vi "TidyOverlappingWiresSubVi.vi"(8 "Error In":errorcluster, 10 "Control references":refnum<vi>[](array[refnum]), 11 "New case structure ref":refnum<vi>) -> (0 "Error Out":errorcluster)   [LabVIEW 2017, in "ErrorStructureDrawer.lvlib"]
doc: "SubVI for tidyOverlappingWires.vi to allow processing of controls and indicators separately."
uses:
  ErrorStructureDrawer.lvlib
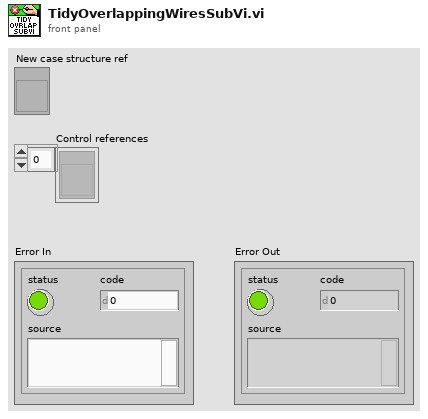
[diagram p1: front panel]
types:
  T1 = typedef "ErrorStructureDrawer.lvlib/ControlConstants.ctl" = cluster{"Half-height of terminal":i32}
  T2 = typedef "LVRectTypeDef.ctl" = cluster{"Left":i16, "Top":i16, "Right":i16, "Bottom":i16}
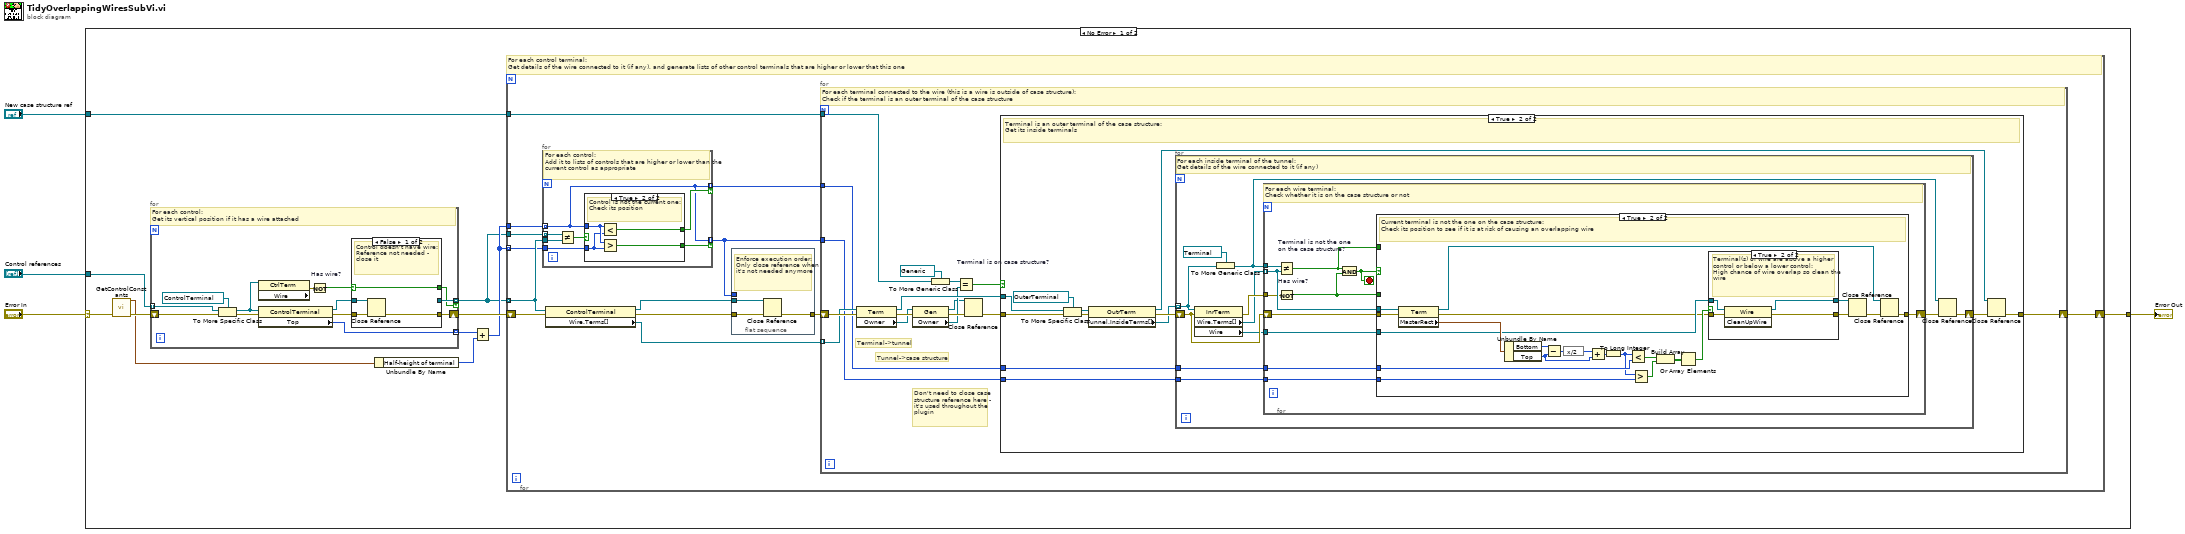
[diagram p0: block diagram]
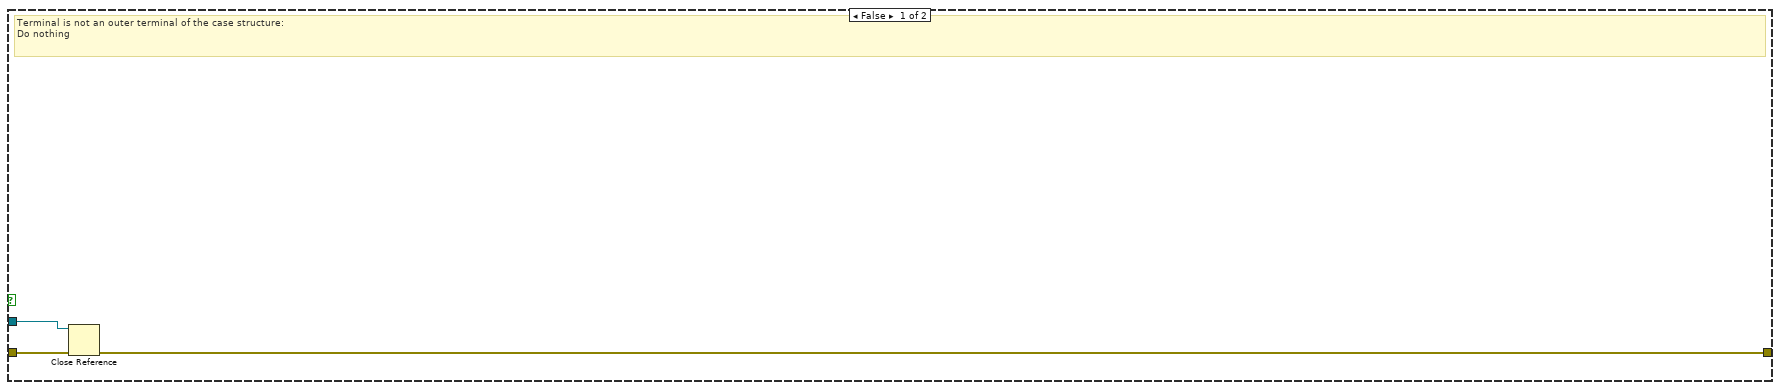
[diagram p3: hidden frame]
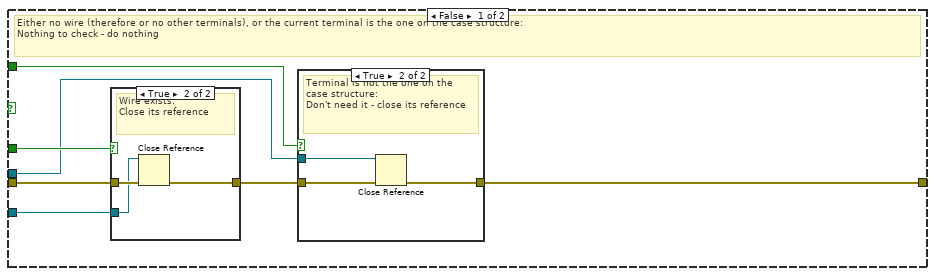
[diagram p4: hidden frame]
diagram:
  n1 = case shown="No Error" "Error In" {
    selector: "Error In" -> [w6 w159]
    tunnel: "Control references" -> [w9 _]
    tunnel: "New case structure ref" -> [w8 _]
    tunnel: [w5 w159] -> w1
    frame No Error {
      n2 = call "GetControlConstants.vi"("error in (no error)"=w6) -> ("error out"=w14:errorcluster, "Control constants"=w7:T1)  [unwired: 9 in]
      n3 = for {
        tunnel: w9 -> [w149] mode=indexing
        tunnel: [w148] -> w11 mode=indexing
        tunnel: [w140] -> w12 mode=indexing if=w139
        shift-right: [w143] -> w15
        shift-left: w14 -> [w147]
        # "For each control:\nGet its vertical position if it has a wire attached"
        n4 = To More Specific Class(target class=refnum<vi> refnum ("New case structure ref"), reference=w149, error in=w147) -> (specific class reference=w144:refnum<vi>, error out=w150:errorcluster)
        n5 = property class="CtrlTerm" props=["Wire"](reference=w144) -> (error out=w145:errorcluster)  [unwired: 1 in, 2 out]
        n6 = property class="ControlTerminal"(reference=w144, error in=w150) -> (reference out=w141:refnum<vi>, error out=w146:errorcluster, "Top"=w148:i32)
        n7 = Not "Has wire?"(x=w145) -> (.not. x?=w142:bool)
        n8 = case shown="False" w142 {
          selector: w142 -> [w152 w157]
          tunnel: w146 -> [w155 w156]
          tunnel: [w154 w156] -> w143
          tunnel: w141 -> [w153 w158]
          tunnel: [_ w158] -> w140
          tunnel: [w152 w157] -> w139
          frame False {
            # "Control doesn't have wire:\nReference not needed - close it"
            n9 = Close Reference(reference=w153, error in (no error)=w155) -> (error out=w154:errorcluster)
          }
          frame True {
            # "Control has wire:\nPass reference through"
          }
        }
      }
      n10 = Unbundle By Name(w7) -> ("Half-height of terminal"=w10:i32)
      n11 = Add(x=w11, y=w10) -> (x+y=w13:i32[])
      n12 = for {
        shift-right: [w22] -> w5
        shift-left: w15 -> [w21]
        tunnel: w8 -> [w26]
        tunnel: w13 -> [w23]
        tunnel: w12 -> [w25]
        tunnel: w12 -> [w20] mode=indexing
        tunnel: w13 -> [w19] mode=indexing
        # "For each control terminal:\nGet details of the wire connected to it (if any), and generate lists of other control terminals that are higher or lower that this one"
        n13 = for {
          tunnel: w23 -> [w33] mode=indexing
          tunnel: w25 -> [w35] mode=indexing
          tunnel: w20 -> [w38]
          tunnel: w19 -> [w36]
          tunnel: [w33] -> w24 mode=indexing if=w34
          tunnel: [w33] -> w16 mode=indexing if=w32
          # "For each control:\nAdd it to lists of controls that are higher or lower than the current control as appropriate"
          n14 = Not Equal?(x=w35, y=w38) -> (x != y?=w37:bool)
          n15 = case shown="True" w37 {
            tunnel: w36 -> [_ w39]
            tunnel: w33 -> [_ w40]
            tunnel: [_ w42] -> w34
            tunnel: [_ w41] -> w32
            frame False {
              # "Control is the current one:\nDo nothing"
            }
            frame True {
              # "Control is not the current one:\nCheck its position"
              n16 = Less?(x=w40, y=w39) -> (x < y?=w42:bool)
              n17 = Greater?(x=w40, y=w39) -> (0:w41:bool)
            }
          }
        }
        n18 = property class="ControlTerminal"(reference=w20, error in=w21) -> (reference out=w17:refnum<vi>, error out=w27:errorcluster, "Wire.Terms[]"=w28:refnum<vi>[])
        n19 = flat-sequence {
          tunnel: w27 -> [w31]
          tunnel: [w30] -> w18
          tunnel: w17 -> [w29]
          tunnel: w16 -> [_]
          frame #0 {
            # "Enforce execution order:\nOnly close reference when it's not needed anymore"
            n20 = Close Reference(reference=w29, error in (no error)=w31) -> (error out=w30:errorcluster)
          }
        }
        n21 = for {
          tunnel: w28 -> [w55] mode=indexing
          shift-right: [w53] -> w22
          shift-left: w18 -> [w56]
          tunnel: w26 -> [w47]
          tunnel: w24 -> [w51]
          tunnel: w16 -> [w50]
          # "Don't need to close case structure reference here - it's used throughout the plugin"
          # "Tunnel->case structure"
          # "Terminal->tunnel"
          # "For each terminal connected to the wire (this is a wire is outside of case structure):\nCheck if the terminal is an outer terminal of the case structure"
          n22 = property class="Term"(reference=w55, error in=w56) -> (reference out=w52:refnum<vi>, error out=w57:errorcluster, "Owner"=w49:refnum<vi>)
          n23 = property class="Gen"(reference=w49, error in=w57) -> (reference out=w43:refnum<vi>, error out=w58:errorcluster, "Owner"=w48:refnum<vi>)
          n24 = To More Generic Class(target class=refnum<vi> refnum ("Owner"), reference=w47) -> (generic class reference=w46:refnum<vi>)
          n25 = Equal? "Terminal is on case structure?"(x=w46, y=w48) -> (x = y?=w54:bool)
          n26 = Close Reference(reference=w43, error in (no error)=w58) -> (error out=w44:errorcluster)
          n27 = case shown="True" w54 {
            tunnel: w44 -> [w61 w72]
            tunnel: [w60 w63] -> w53
            tunnel: w52 -> [w59 w71]
            tunnel: w51 -> [_ w65]
            tunnel: w50 -> [_ w64]
            frame False {
              # "Terminal is not an outer terminal of the case structure:\nDo nothing"
              n28 = Close Reference(reference=w59, error in (no error)=w61) -> (error out=w60:errorcluster)
            }
            frame True {
              # "Terminal is an outer terminal of the case structure:\nGet its inside terminals"
              n29 = To More Specific Class(target class=refnum<vi> refnum ("Outside Terminal"), reference=w71, error in=w72) -> (specific class reference=w69:refnum<vi>, error out=w68:errorcluster)
              n30 = property class="OutrTerm"(reference=w69, error in=w68) -> (reference out=w62:refnum<vi>, error out=w73:errorcluster, "Tunnel.InsideTerms[]"=w67:refnum<vi>[])
              n31 = for {
                tunnel: w67 -> [w77] mode=indexing
                shift-right: [w75] -> w66
                shift-left: w73 -> [w83]
                tunnel: w65 -> [w80]
                tunnel: w64 -> [w79]
                # "For each inside terminal of the tunnel:\nGet details of the wire connected to it (if any)"
                n32 = property class="InrTerm"(reference=w77, error in=w83) -> (error out=w84:errorcluster, "Wire.Terms[]"=w82:refnum<vi>[], "Wire"=w78:refnum<vi>)  [unwired: 1 out]
                n33 = To More Generic Class(target class=refnum<vi> refnum ("element"), reference=w77) -> (generic class reference=w74:refnum<vi>)
                n34 = for {
                  tunnel: w82 -> [w92] mode=indexing
                  tunnel: w74 -> [w95]
                  shift-right: [w93] -> w81
                  shift-left: w83 -> [w94]
                  tunnel: w80 -> [w91]
                  tunnel: w79 -> [w90]
                  tunnel: w78 -> [w89]
                  tunnel: w84 -> [w88]
                  stop <- w87 stop-if-true
                  # "For each wire terminal:\nCheck whether it is on the case structure or not"
                  n35 = Not Equal? "Terminal is not the one on the case structure?"(x=w95, y=w92) -> (x != y?=w85:bool)
                  n36 = Not "Has wire?"(x=w88) -> (.not. x?=w86:bool)
                  n37 = And(x=w85, y=w86) -> (x .and. y?=w87:bool)
                  n38 = case shown="True" w87 {
                    tunnel: w94 -> [w102 w132]
                    tunnel: [w98 w112] -> w93
                    tunnel: w92 -> [w97 w131]
                    tunnel: w91 -> [_ w127]
                    tunnel: w90 -> [_ w126]
                    tunnel: w89 -> [w100 w120]
                    tunnel: w86 -> [w99 _]
                    tunnel: w85 -> [w96 _]
                    frame False {
                      # "Either no wire (therefore or no other terminals), or the current terminal is the one on the case structure:\nNothing to check - do nothing"
                      n39 = case shown="True" w99 {
                        tunnel: w102 -> [w107 w110]
                        tunnel: [w107 w109] -> w101
                        tunnel: w100 -> [_ w108]
                        frame False {
                          # "No wire:\nDo nothing"
                        }
                        frame True {
                          # "Wire exists:\nClose its reference"
                          n40 = Close Reference(reference=w108, error in (no error)=w110) -> (error out=w109:errorcluster)
                        }
                      }
                      n41 = case shown="True" w96 {
                        tunnel: w101 -> [w103 w106]
                        tunnel: [w103 w105] -> w98
                        tunnel: w97 -> [_ w104]
                        frame False {
                          # "Terminal is the one on the case structure:\nDo nothing"
                        }
                        frame True {
                          # "Terminal is not the one on the case structure:\nDon't need it - close its reference"
                          n42 = Close Reference(reference=w104, error in (no error)=w106) -> (error out=w105:errorcluster)
                        }
                      }
                    }
                    frame True {
                      # "Current terminal is not the one on the case structure:\nCheck its position to see if it is at risk of causing an overlapping wire"
                      n43 = property class="Term"(reference=w131, error in=w132) -> (reference out=w111:refnum<vi>, error out=w113:errorcluster, "MasterRect"=w130:T2)
                      n44 = Unbundle By Name(w130) -> ("Bottom"=w129:i16, "Top"=w118:i16)
                      n45 = Subtract(x=w129, y=w118) -> (x-y=w128:i16)
                      n46 = expression code="x/2"(w128) -> (w119:i16)
                      n47 = Add(x=w119, y=w118) -> (x+y=w117:i16)
                      n48 = To Long Integer(number=w117) -> (32bit integer=w116:i32)
                      n49 = Less?(x=w116, y=w127) -> (x < y?=w125:bool[])
                      n50 = Greater?(x=w116, y=w126) -> (0:w124:bool[])
                      n51 = Build Array(w125, w124) -> (w123:bool[][])
                      n52 = Or Array Elements(Boolean array=w123) -> (logical OR=w122:bool)
                      n53 = case shown="True" w122 {
                        tunnel: w113 -> [w134 w138]
                        tunnel: [w134 w137] -> w121
                        tunnel: w120 -> [w133 w136]
                        tunnel: [w133 w135] -> w114
                        frame False {
                          # "No terminal(s) of wire are above a higher control or below a lower control:\nLower chance of wire overlap so do nothing"
                        }
                        frame True {
                          # "Terminal(s) of wire are above a higher control or below a lower control:\nHigh chance of wire overlap so clean the wire"
                          n54 = invoke class="Wire" method="CleanUpWire"(reference=w136, error in=w138) -> (reference out=w135:refnum<vi>, error out=w137:errorcluster)  [unwired: 1 in, 1 out]
                        }
                      }
                      n55 = Close Reference(reference=w114, error in (no error)=w121) -> (error out=w115:errorcluster)
                      n56 = Close Reference(reference=w111, error in (no error)=w115) -> (error out=w112:errorcluster)
                    }
                  }
                }
                n57 = Close Reference(reference=w74, error in (no error)=w81) -> (error out=w75:errorcluster)
              }
              n58 = Close Reference(reference=w62, error in (no error)=w66) -> (error out=w63:errorcluster)
            }
          }
        }
      }
    }
    frame Error {
    }
  }
  "Error Out" <- w1
